vi "LS370_only_readout_Monitor.vi"() -> ()   [LabVIEW 2019]
uses:
  Utility/LS370/Monitor/LS370_only_readout_cluster.ctl
  Instrument_Setup.vi
  Global/Global Variables/Data_Display_global.vi
panel:
  out "Lakeshore 370 read only":T1
  in  "error in (no error)":errorcluster
  in  "Stopp":bool
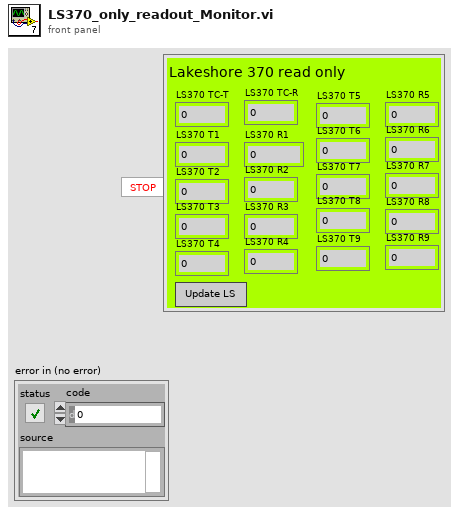
[diagram p1: front panel]
types:
  T1 = typedef "LS370_only_readout_cluster.ctl" = cluster{"LS370 T1":dbl, "LS370 T2":dbl, "LS370 T3":dbl, "LS370 T4":dbl, "LS370 T5":dbl, "LS370 R1":dbl, "LS370 R2":dbl, "LS370 R3":dbl, "LS370 R4":dbl, "LS370 R5":dbl, "LS370 T6":dbl, "LS370 T7":dbl, "LS370 T8":dbl, "LS370 T9":dbl, "LS370 R6":dbl, "LS370 R7":dbl, "LS370 R8":dbl, "LS370 R9":dbl, "LS370 TC-T":dbl, "LS370 TC-R":dbl, "Update Lakeshores":bool}
  T2 = typedef "LS370_read_only_control.ctl" = cluster{"Update Lakeshores":bool}
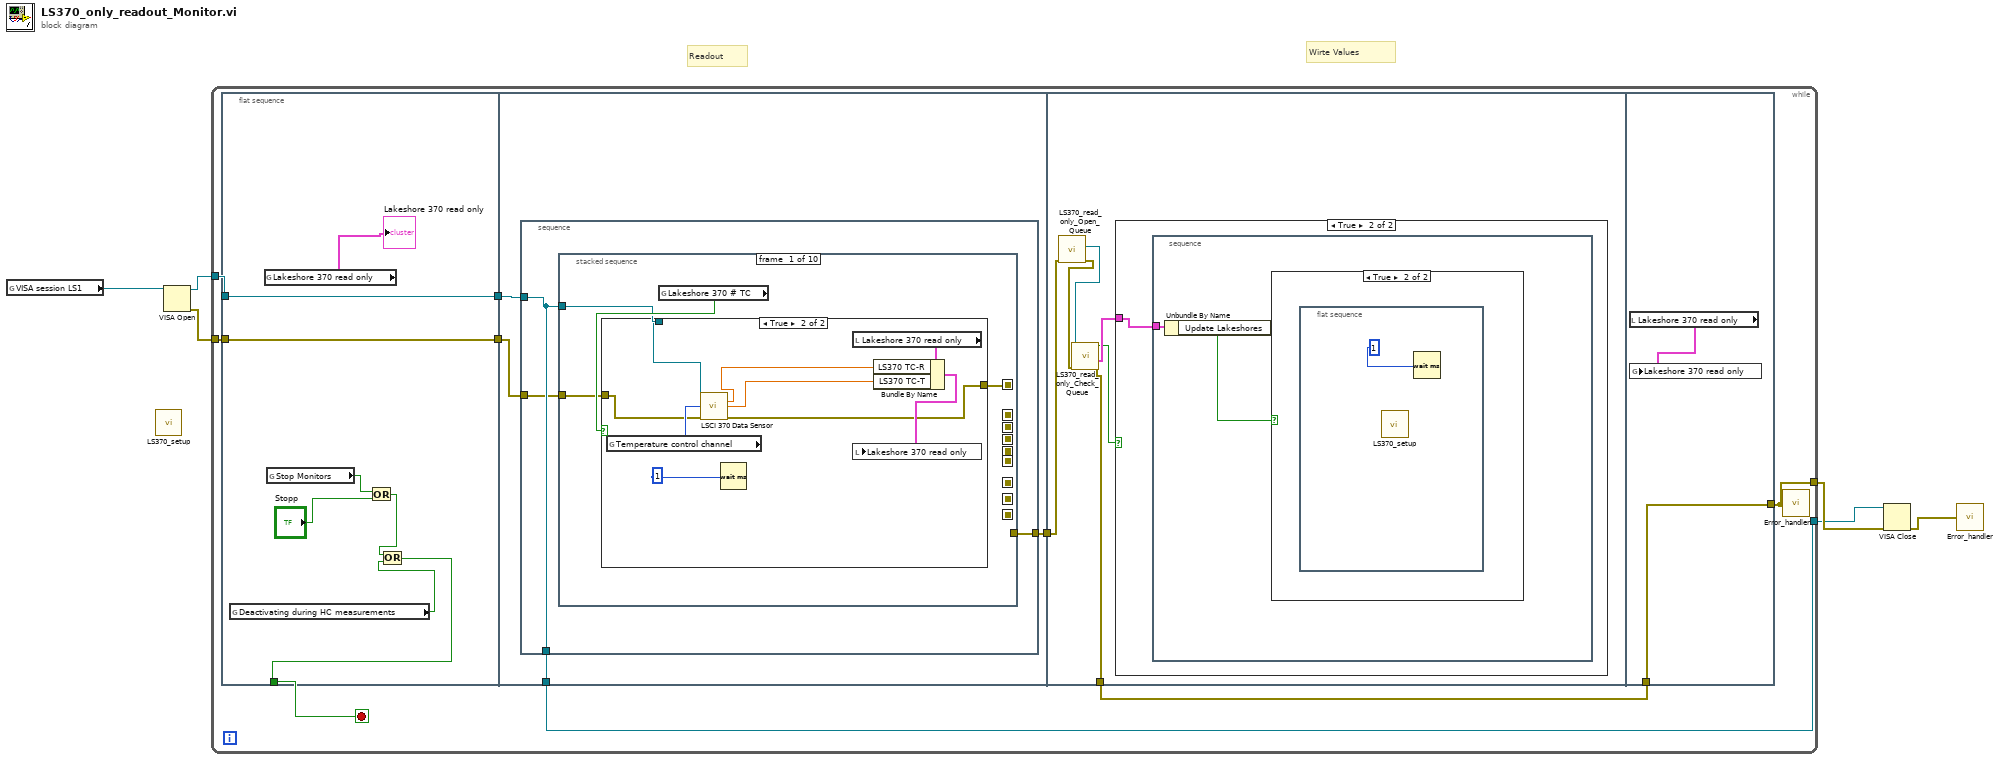
[diagram p0: block diagram]
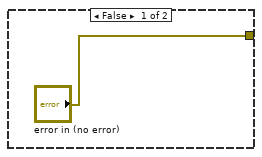
[diagram p2: hidden frame]
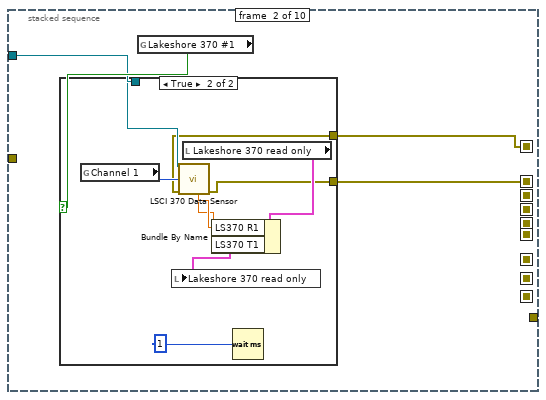
[diagram p3: hidden frame]
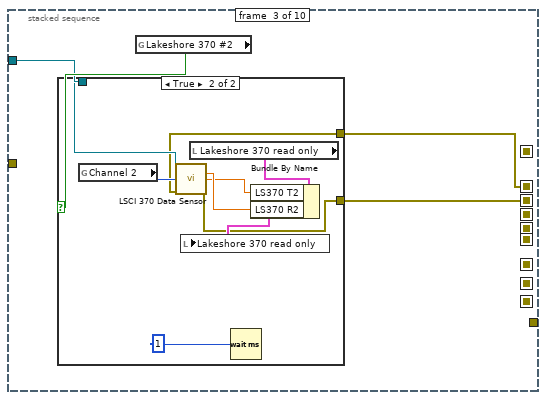
[diagram p5: hidden frame]
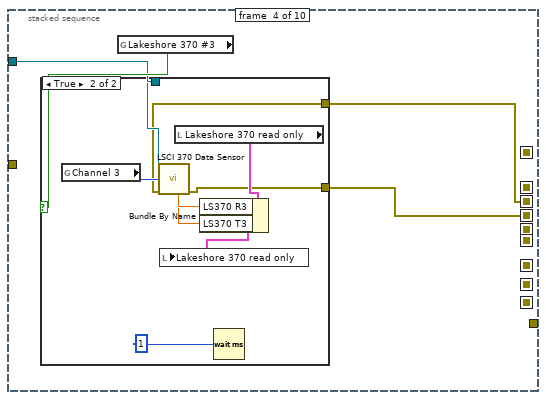
[diagram p7: hidden frame]
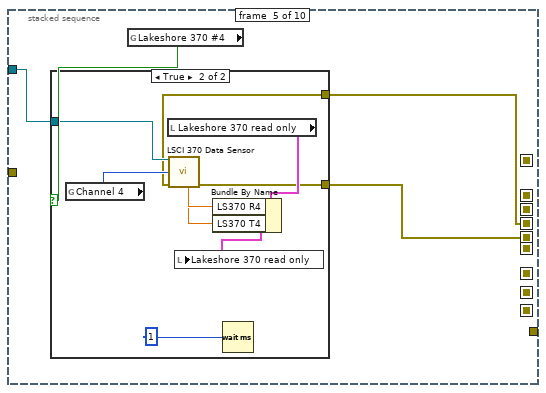
[diagram p9: hidden frame]
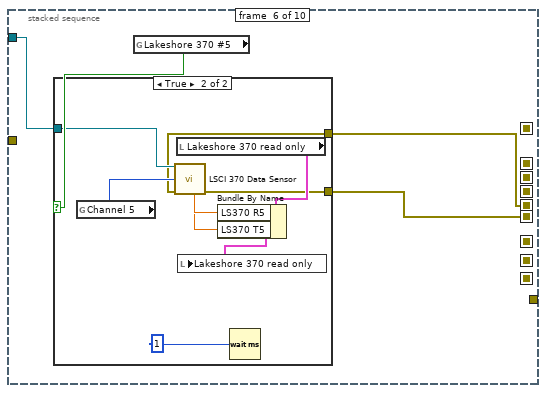
[diagram p11: hidden frame]
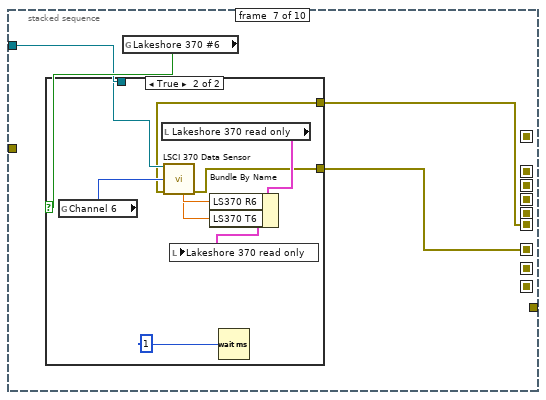
[diagram p13: hidden frame]
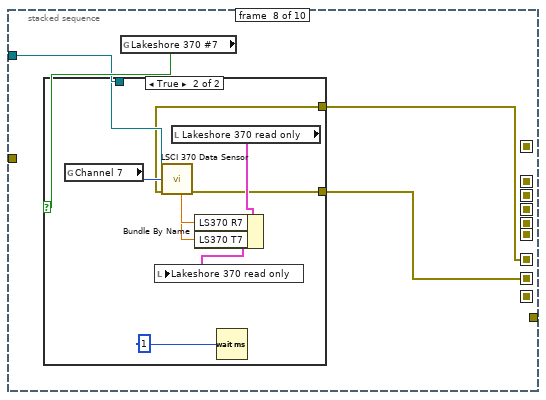
[diagram p15: hidden frame]
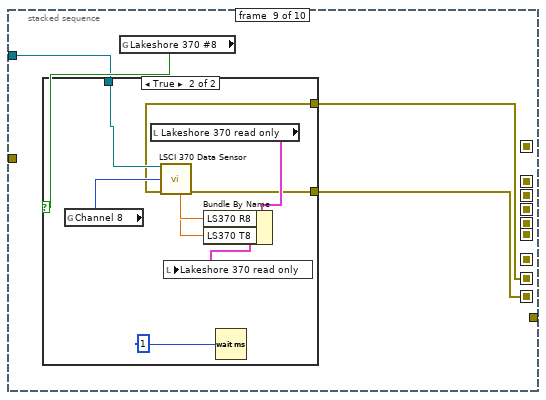
[diagram p17: hidden frame]
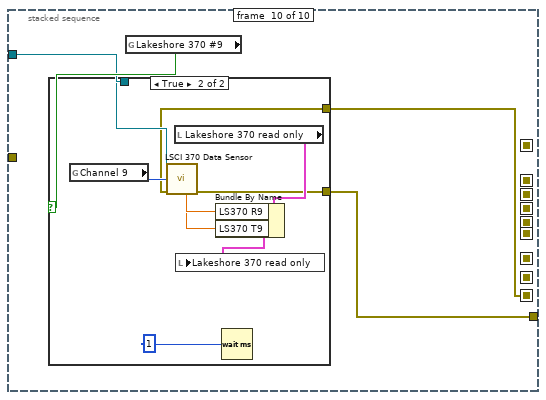
[diagram p19: hidden frame]
diagram:
  # "Wirte Values"
  # "Readout"
  n1 = global read "Instrument_Setup.vi" "VISA session LS1"() -> (w3:refnum<visa-resource-name>)
  n2 = call "LS370_setup.vi"() -> ()  [unwired: 1 in]
  n3 = VISA Open(VISA resource name=w3) -> (VISA resource name=w2:refnum<visa-resource-name>, error out=w1:errorcluster)  [unwired: 4 in]
  n4 = while {
    tunnel: w2 -> [w14]
    tunnel: [w10] -> w6
    tunnel: [w9] -> w5
    tunnel: w1 -> [w7]
    stop <- w13 stop-if-true
    n5 = flat-sequence {
      tunnel: w14 -> [w23]
      tunnel: [w23] -> w15
      tunnel: [w22] -> w13
      tunnel: [w20] -> w8
      tunnel: w7 -> [w20]
      tunnel: w15 -> [w27]
      tunnel: [w26] -> w12
      tunnel: [w25] -> w9
      tunnel: w8 -> [w24]
      tunnel: w12 -> [w173]
      tunnel: [w171] -> w11
      tunnel: w11 -> [w181]
      tunnel: [w181] -> w10
      frame #0 {
        n6 = global read "Data_Display_global.vi" "Deactivating during HC measurements"() -> (w16:bool)
        n7 = global read "Data_Display_global.vi" "Lakeshore 370 read only"() -> (→"Lakeshore 370 read only":T1)
        n8 = global read "Data_Display_global.vi" "Stop Monitors"() -> (w19:bool)
        n9 = Or(x=w19, y="Stopp") -> (x .or. y?=w17:bool)
        n10 = Or(x=w17, y=w16) -> (x .or. y?=w22:bool)
      }
      frame #1 {
        n11 = stacked-sequence {
          tunnel: w27 -> [w29]
          tunnel: [w30] -> w26
          tunnel: [w29] -> w25
          tunnel: w24 -> [w28]
          frame #0 {
            n12 = stacked-sequence {
              seq-local: [w32 _ _ _ _ _ _ _ _ _] -> [_ w46 _ _ _ _ _ _ _ _]
              seq-local: [_ w45 _ _ _ _ _ _ _ _] -> [_ _ w60 _ _ _ _ _ _ _]
              seq-local: [_ _ w59 _ _ _ _ _ _ _] -> [_ _ _ w74 _ _ _ _ _ _]
              seq-local: [_ _ _ w73 _ _ _ _ _ _] -> [_ _ _ _ w88 _ _ _ _ _]
              seq-local: [_ _ _ _ w87 _ _ _ _ _] -> [_ _ _ _ _ w102 _ _ _ _]
              seq-local: [_ _ _ _ _ w101 _ _ _ _] -> [_ _ _ _ _ _ w116 _ _ _]
              seq-local: [_ _ _ _ _ _ w115 _ _ _] -> [_ _ _ _ _ _ _ w130 _ _]
              seq-local: [_ _ _ _ _ _ _ w129 _ _] -> [_ _ _ _ _ _ _ _ w144 _]
              seq-local: [_ _ _ _ _ _ _ _ w143 _] -> [_ _ _ _ _ _ _ _ _ w158]
              tunnel: w29 -> [w33 w47 w61 w75 w89 w103 w117 w131 w145 w159]
              tunnel: [_ _ _ _ _ _ _ _ _ w157] -> w30
              tunnel: w28 -> [w31 _ _ _ _ _ _ _ _ _]
              frame #0 {
                n13 = global read "Instrument_Setup.vi" "Lakeshore 370 # TC"() -> (w34:bool)
                n14 = case shown="True" w34 {
                  tunnel: w33 -> [_ w42]
                  tunnel: ["error in (no error)" w37] -> w32
                  tunnel: w31 -> [_ w36]
                  frame False {
                  }
                  frame True {
                    n15 = global read "Instrument_Setup.vi" "Temperature control channel"() -> (w44:i32)
                    n16 = call "LSCI 370 Data Sensor.vi"("VISA session"=w42, "Channel (1)"=w44, "error in (no error)"=w36) -> ("Resistance Reading"=w40:dbl, "Kelvin Reading"=w39:dbl, "error out"=w37:errorcluster)  [unwired: 8 in, 2 out]
                    n17 = Wait (ms)(milliseconds to wait=1) -> ()  [unwired: 1 out]
                    n18 = local read "Lakeshore 370 read only"() -> (w41:T1)
                    n19 = Bundle By Name(cluster=w41, "LS370 TC-R"=w40, "LS370 TC-T"=w39) -> (w38:T1)
                    n20 = local write "Lakeshore 370 read only"(w38) -> ()
                  }
                }
              }
              frame #1 {
                n21 = global read "Instrument_Setup.vi" "Lakeshore 370 #1"() -> (w48:bool)
                n22 = case shown="True" w48 {
                  tunnel: w47 -> [_ w56]
                  tunnel: w46 -> [w49 w51]
                  tunnel: [w49 w50] -> w45
                  frame False {
                  }
                  frame True {
                    n23 = global read "Instrument_Setup.vi" "Channel 1"() -> (w58:i32)
                    n24 = call "LSCI 370 Data Sensor.vi"("VISA session"=w56, "Channel (1)"=w58, "error in (no error)"=w51) -> ("Resistance Reading"=w53:dbl, "Kelvin Reading"=w52:dbl, "error out"=w50:errorcluster)  [unwired: 8 in, 2 out]
                    n25 = local read "Lakeshore 370 read only"() -> (w55:T1)
                    n26 = Bundle By Name(cluster=w55, "LS370 R1"=w53, "LS370 T1"=w52) -> (w54:T1)
                    n27 = local write "Lakeshore 370 read only"(w54) -> ()
                    n28 = Wait (ms)(milliseconds to wait=1) -> ()  [unwired: 1 out]
                  }
                }
              }
              frame #2 {
                n29 = global read "Instrument_Setup.vi" "Lakeshore 370 #2"() -> (w62:bool)
                n30 = case shown="True" w62 {
                  tunnel: w61 -> [_ w70]
                  tunnel: w60 -> [w63 w65]
                  tunnel: [w63 w64] -> w59
                  frame False {
                  }
                  frame True {
                    n31 = global read "Instrument_Setup.vi" "Channel 2"() -> (w72:i32)
                    n32 = call "LSCI 370 Data Sensor.vi"("VISA session"=w70, "Channel (1)"=w72, "error in (no error)"=w65) -> ("Resistance Reading"=w67:dbl, "Kelvin Reading"=w66:dbl, "error out"=w64:errorcluster)  [unwired: 8 in, 2 out]
                    n33 = local read "Lakeshore 370 read only"() -> (w69:T1)
                    n34 = Wait (ms)(milliseconds to wait=1) -> ()  [unwired: 1 out]
                    n35 = Bundle By Name(cluster=w69, "LS370 T2"=w66, "LS370 R2"=w67) -> (w68:T1)
                    n36 = local write "Lakeshore 370 read only"(w68) -> ()
                  }
                }
              }
              frame #3 {
                n37 = global read "Instrument_Setup.vi" "Lakeshore 370 #3"() -> (w76:bool)
                n38 = case shown="True" w76 {
                  tunnel: w75 -> [_ w84]
                  tunnel: w74 -> [w77 w79]
                  tunnel: [w77 w78] -> w73
                  frame False {
                  }
                  frame True {
                    n39 = global read "Instrument_Setup.vi" "Channel 3"() -> (w86:i32)
                    n40 = call "LSCI 370 Data Sensor.vi"("VISA session"=w84, "Channel (1)"=w86, "error in (no error)"=w79) -> ("Resistance Reading"=w81:dbl, "Kelvin Reading"=w80:dbl, "error out"=w78:errorcluster)  [unwired: 8 in, 2 out]
                    n41 = local read "Lakeshore 370 read only"() -> (w83:T1)
                    n42 = Bundle By Name(cluster=w83, "LS370 R3"=w81, "LS370 T3"=w80) -> (w82:T1)
                    n43 = local write "Lakeshore 370 read only"(w82) -> ()
                    n44 = Wait (ms)(milliseconds to wait=1) -> ()  [unwired: 1 out]
                  }
                }
              }
              frame #4 {
                n45 = global read "Instrument_Setup.vi" "Lakeshore 370 #4"() -> (w90:bool)
                n46 = case shown="True" w90 {
                  tunnel: w89 -> [_ w98]
                  tunnel: w88 -> [w91 w93]
                  tunnel: [w91 w92] -> w87
                  frame False {
                  }
                  frame True {
                    n47 = global read "Instrument_Setup.vi" "Channel 4"() -> (w100:i32)
                    n48 = local read "Lakeshore 370 read only"() -> (w97:T1)
                    n49 = call "LSCI 370 Data Sensor.vi"("VISA session"=w98, "Channel (1)"=w100, "error in (no error)"=w93) -> ("Resistance Reading"=w95:dbl, "Kelvin Reading"=w94:dbl, "error out"=w92:errorcluster)  [unwired: 8 in, 2 out]
                    n50 = Bundle By Name(cluster=w97, "LS370 R4"=w95, "LS370 T4"=w94) -> (w96:T1)
                    n51 = local write "Lakeshore 370 read only"(w96) -> ()
                    n52 = Wait (ms)(milliseconds to wait=1) -> ()  [unwired: 1 out]
                  }
                }
              }
              frame #5 {
                n53 = global read "Instrument_Setup.vi" "Lakeshore 370 #5"() -> (w104:bool)
                n54 = case shown="True" w104 {
                  tunnel: w103 -> [_ w112]
                  tunnel: w102 -> [w105 w107]
                  tunnel: [w105 w106] -> w101
                  frame False {
                  }
                  frame True {
                    n55 = global read "Instrument_Setup.vi" "Channel 5"() -> (w114:i32)
                    n56 = call "LSCI 370 Data Sensor.vi"("VISA session"=w112, "Channel (1)"=w114, "error in (no error)"=w107) -> ("Resistance Reading"=w110:dbl, "Kelvin Reading"=w109:dbl, "error out"=w106:errorcluster)  [unwired: 8 in, 2 out]
                    n57 = local read "Lakeshore 370 read only"() -> (w111:T1)
                    n58 = Bundle By Name(cluster=w111, "LS370 R5"=w110, "LS370 T5"=w109) -> (w108:T1)
                    n59 = local write "Lakeshore 370 read only"(w108) -> ()
                    n60 = Wait (ms)(milliseconds to wait=1) -> ()  [unwired: 1 out]
                  }
                }
              }
              frame #6 {
                n61 = global read "Instrument_Setup.vi" "Lakeshore 370 #6"() -> (w118:bool)
                n62 = case shown="True" w118 {
                  tunnel: w117 -> [_ w126]
                  tunnel: w116 -> [w119 w121]
                  tunnel: [w119 w120] -> w115
                  frame False {
                  }
                  frame True {
                    n63 = global read "Instrument_Setup.vi" "Channel 6"() -> (w128:i32)
                    n64 = local read "Lakeshore 370 read only"() -> (w125:T1)
                    n65 = call "LSCI 370 Data Sensor.vi"("VISA session"=w126, "Channel (1)"=w128, "error in (no error)"=w121) -> ("Resistance Reading"=w124:dbl, "Kelvin Reading"=w123:dbl, "error out"=w120:errorcluster)  [unwired: 8 in, 2 out]
                    n66 = Bundle By Name(cluster=w125, "LS370 R6"=w124, "LS370 T6"=w123) -> (w122:T1)
                    n67 = local write "Lakeshore 370 read only"(w122) -> ()
                    n68 = Wait (ms)(milliseconds to wait=1) -> ()  [unwired: 1 out]
                  }
                }
              }
              frame #7 {
                n69 = global read "Instrument_Setup.vi" "Lakeshore 370 #7"() -> (w132:bool)
                n70 = case shown="True" w132 {
                  tunnel: w131 -> [_ w140]
                  tunnel: w130 -> [w133 w135]
                  tunnel: [w133 w134] -> w129
                  frame False {
                  }
                  frame True {
                    n71 = global read "Instrument_Setup.vi" "Channel 7"() -> (w142:i32)
                    n72 = call "LSCI 370 Data Sensor.vi"("VISA session"=w140, "Channel (1)"=w142, "error in (no error)"=w135) -> ("Resistance Reading"=w138:dbl, "Kelvin Reading"=w137:dbl, "error out"=w134:errorcluster)  [unwired: 8 in, 2 out]
                    n73 = local read "Lakeshore 370 read only"() -> (w139:T1)
                    n74 = Bundle By Name(cluster=w139, "LS370 R7"=w138, "LS370 T7"=w137) -> (w136:T1)
                    n75 = local write "Lakeshore 370 read only"(w136) -> ()
                    n76 = Wait (ms)(milliseconds to wait=1) -> ()  [unwired: 1 out]
                  }
                }
              }
              frame #8 {
                n77 = global read "Instrument_Setup.vi" "Lakeshore 370 #8"() -> (w146:bool)
                n78 = case shown="True" w146 {
                  tunnel: w145 -> [_ w154]
                  tunnel: w144 -> [w147 w149]
                  tunnel: [w147 w148] -> w143
                  frame False {
                  }
                  frame True {
                    n79 = global read "Instrument_Setup.vi" "Channel 8"() -> (w156:i32)
                    n80 = local read "Lakeshore 370 read only"() -> (w153:T1)
                    n81 = call "LSCI 370 Data Sensor.vi"("VISA session"=w154, "Channel (1)"=w156, "error in (no error)"=w149) -> ("Resistance Reading"=w152:dbl, "Kelvin Reading"=w151:dbl, "error out"=w148:errorcluster)  [unwired: 8 in, 2 out]
                    n82 = Bundle By Name(cluster=w153, "LS370 R8"=w152, "LS370 T8"=w151) -> (w150:T1)
                    n83 = local write "Lakeshore 370 read only"(w150) -> ()
                    n84 = Wait (ms)(milliseconds to wait=1) -> ()  [unwired: 1 out]
                  }
                }
              }
              frame #9 {
                n85 = global read "Instrument_Setup.vi" "Lakeshore 370 #9"() -> (w160:bool)
                n86 = case shown="True" w160 {
                  tunnel: w159 -> [_ w168]
                  tunnel: w158 -> [w161 w163]
                  tunnel: [w161 w162] -> w157
                  frame False {
                  }
                  frame True {
                    n87 = global read "Instrument_Setup.vi" "Channel 9"() -> (w170:i32)
                    n88 = call "LSCI 370 Data Sensor.vi"("VISA session"=w168, "Channel (1)"=w170, "error in (no error)"=w163) -> ("Resistance Reading"=w166:dbl, "Kelvin Reading"=w165:dbl, "error out"=w162:errorcluster)  [unwired: 8 in, 2 out]
                    n89 = local read "Lakeshore 370 read only"() -> (w167:T1)
                    n90 = Bundle By Name(cluster=w167, "LS370 R9"=w166, "LS370 T9"=w165) -> (w164:T1)
                    n91 = local write "Lakeshore 370 read only"(w164) -> ()
                    n92 = Wait (ms)(milliseconds to wait=1) -> ()  [unwired: 1 out]
                  }
                }
              }
            }
          }
        }
      }
      frame #2 {
        n93 = call "LS370_read_only_Open_Queue.vi"("error in (no error)"=w173) -> ("error out"=w172:errorcluster, "queue out"=w175:refnum<queue>)  [unwired: 9 in]
        n94 = call "LS370_read_only_Check_Queue.vi"("error in (no error)"=w172, "queue"=w175) -> ("error out"=w171:errorcluster, "Lakeshore 370 read only Control"=w176:T2, "New Entries?"=w174:bool)  [unwired: 6 in]
        n95 = case shown="True" w174 {
          tunnel: w176 -> [_ w177]
          frame False {
          }
          frame True {
            n96 = stacked-sequence {
              tunnel: w177 -> [w179]
              frame #0 {
                n97 = Unbundle By Name(w179) -> ("Update Lakeshores"=w178:bool)
                n98 = case shown="True" w178 {
                  frame False {
                  }
                  frame True {
                    n99 = flat-sequence {
                      frame #0 {
                        n100 = call "LS370_setup.vi"() -> ()  [unwired: 1 in]
                        n101 = Wait (ms)(milliseconds to wait=1) -> ()  [unwired: 1 out]
                      }
                    }
                  }
                }
              }
            }
          }
        }
      }
      frame #3 {
        n102 = local read "Lakeshore 370 read only"() -> (w182:T1)
        n103 = global write "Data_Display_global.vi" "Lakeshore 370 read only"(w182) -> ()
      }
    }
    n104 = call "Error_handler.vi"("error constant"=w10) -> ()
  }
  n105 = VISA Close(VISA resource name=w5, error in (no error)=w6) -> (error out=w4:errorcluster)
  n106 = call "Error_handler.vi"("error constant"=w4) -> ()
